vi "GetIndexFromComboCtrl.vi"(10 "search":string, 11 "enum ref":refnum<vi>) -> (3 "index":i32)   [LabVIEW 2018, in "Library-Ctrl.lvlib"]
uses:
  Library-Ctrl.lvlib
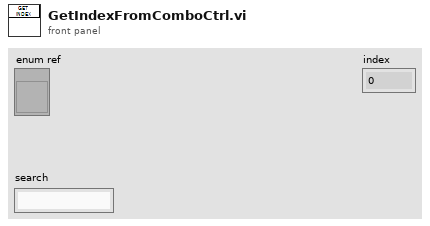
[diagram p1: front panel]
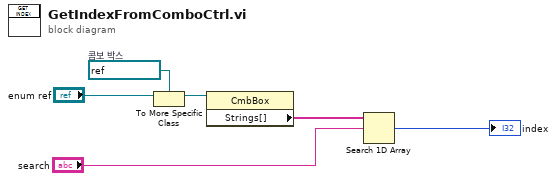
[diagram p0: block diagram]
diagram:
  w5 = refnum<vi> refnum  # 콤보 박스
  n1 = To More Specific Class(target class=w5, reference="enum ref") -> (specific class reference=w4:refnum<vi>)  [unwired: 1 in, 1 out]
  n2 = property class="CmbBox"(reference=w4) -> ("Strings[]"=w3:string[])  [unwired: 1 in, 2 out]
  n3 = Search 1D Array(1D array=w3, element="search") -> (index of element=→"index":i32)  [unwired: 1 in]
